vi "train berth.vi"() -> ()   [LabVIEW 2018]
panel:
  out "SEAT AVAILABILITY":bool
  out "String":string
  in  "Numeric":u8
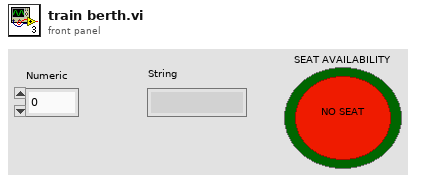
[diagram p1: front panel]
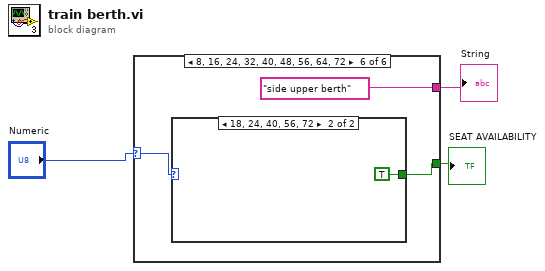
[diagram p0: block diagram]
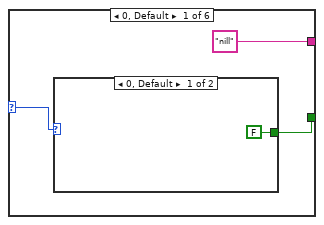
[diagram p2: hidden frame]
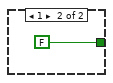
[diagram p3: hidden frame]
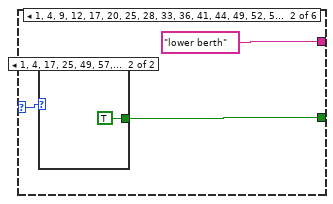
[diagram p4: hidden frame]
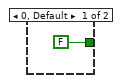
[diagram p5: hidden frame]
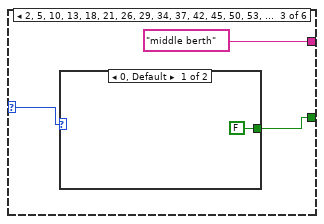
[diagram p6: hidden frame]
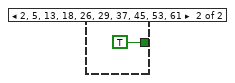
[diagram p7: hidden frame]
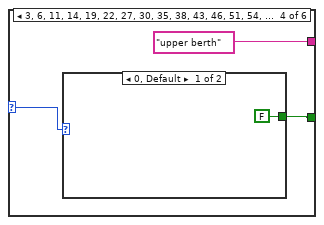
[diagram p8: hidden frame]
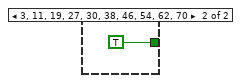
[diagram p9: hidden frame]
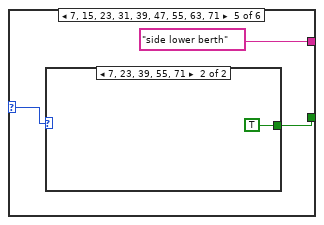
[diagram p10: hidden frame]
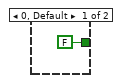
[diagram p11: hidden frame]
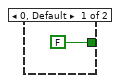
[diagram p12: hidden frame]
diagram:
  n1 = case shown="8, 16, 24, 32, 40, 48, 56, 64, 72" "Numeric" {
    selector: "Numeric" -> [w5 w10 w15 w20 w25 w30]
    tunnel: ["nill" "lower berth" "middle berth" "upper berth" "side lower berth" "side upper berth"] -> w2
    tunnel: [w4 w9 w14 w19 w24 w29] -> w1
    frame 0, Default {
      n2 = case shown="0, Default" w5 {
        tunnel: [FALSE FALSE] -> w4
        frame 0, Default {
        }
        frame 1 {
        }
      }
    }
    frame 1, 4, 9, 12, 17, 20, 25, 28, 33, 36, 41, 44, 49, 52, 57, 60, 65, 68 {
      n3 = case shown="1, 4, 17, 25, 49, 57, 65" w10 {
        tunnel: [FALSE TRUE] -> w9
        frame 0, Default {
        }
        frame 1, 4, 17, 25, 49, 57, 65 {
        }
      }
    }
    frame 2, 5, 10, 13, 18, 21, 26, 29, 34, 37, 42, 45, 50, 53, 58, 61, 66, 69 {
      n4 = case shown="0, Default" w15 {
        tunnel: [FALSE TRUE] -> w14
        frame 0, Default {
        }
        frame 2, 5, 13, 18, 26, 29, 37, 45, 53, 61 {
        }
      }
    }
    frame 3, 6, 11, 14, 19, 22, 27, 30, 35, 38, 43, 46, 51, 54, 59, 62, 67, 70 {
      n5 = case shown="0, Default" w20 {
        tunnel: [FALSE TRUE] -> w19
        frame 0, Default {
        }
        frame 3, 11, 19, 27, 30, 38, 46, 54, 62, 70 {
        }
      }
    }
    frame 7, 15, 23, 31, 39, 47, 55, 63, 71 {
      n6 = case shown="7, 23, 39, 55, 71" w25 {
        tunnel: [FALSE TRUE] -> w24
        frame 0, Default {
        }
        frame 7, 23, 39, 55, 71 {
        }
      }
    }
    frame 8, 16, 24, 32, 40, 48, 56, 64, 72 {
      n7 = case shown="18, 24, 40, 56, 72" w30 {
        tunnel: [FALSE TRUE] -> w29
        frame 0, Default {
        }
        frame 18, 24, 40, 56, 72 {
        }
      }
    }
  }
  "String" <- w2
  "SEAT AVAILABILITY" <- w1
